vi "CubeLiftOutput.vi"   [LabVIEW 2017]
uses:
  CubeLiftOutput.ctl
  <vilib>/Rock Robotics/WPI/ThirdParty/Phoenix-LabVIEW/Motor Controller/Controls/CTRE_Phoenix_MotorControl_ControlMode.ctl
  <vilib>/Rock Robotics/WPI/Solenoid/WPI_SolenoidValue.ctl
  <vilib>/Rock Robotics/WPI/Solenoid/WPI_SolenoidSetEnum.vi
types:
  T1 = typedef "CubeLiftOutput.ctl" = cluster{"LiftOutputSetting":dbl, "DepositCube?":bool, "LiftControlMode":T2}
  T2 = typedef "CTRE_Phoenix_MotorControl_ControlMode.ctl" = u16
  T3 = typedef "WPI_SolenoidValue.ctl" = enum16{"Off", "On", "Forward", "Reverse"}
  T4 = typedef "WPI_MotorControlDeviceRef.ctl" = cluster{"DeviceStatus":errorcluster, "Type":T5, "PWM":cluster{"PWM Channel":T6, "DeadBand":T7}, "CAN":cluster{"Device Number":u8, "SetOutput VI Ref":variant, "GetOutput VI Ref":variant, "Enable VI Ref":variant, "Disable VI Ref":variant, "Data":variant}, "Invert":bool, "DIO PWM":cluster{"PWM \"Enable\" Channel":T6, "DIOChannel":T8, "PWM Rate":dbl}}
  T5 = typedef "WPI_MotorControlType.ctl" = enum16{"PWM", "CAN", "DIO PWM"}
  T6 = typedef "FPGA_DIOPWMChannel.ctl" = enum8{"PWM 0", "PWM 1", "PWM 2", "PWM 3", "PWM 4", "PWM 5", "PWM 6", "PWM 7", "PWM 8", "PWM 9", "PWM MXP 0", "PWM MXP 1", "PWM MXP 2", "PWM MXP 3", "PWM MXP 4", "PWM MXP 5", "PWM MXP 6", "PWM MXP 7", "PWM MXP 8", "PWM MXP 9", "Invalid"}
  T7 = typedef "WPI_PWMDeadband.ctl" = cluster{"Name":string, "maxPositivePwm":i32, "minPositivePwm":i32, "centerPwm":i32, "maxNegativePwm":i32, "minNegativePwm":i32, "angularRange":u16}
  T8 = typedef "FPGA_DIOChannel.ctl" = enum8{"DIO 0", "DIO 1", "DIO 2", "DIO 3", "DIO 4", "DIO 5", "DIO 6", "DIO 7", "DIO 8", "DIO 9", "DIO MXP 0", "DIO MXP 1", "DIO MXP 2", "DIO MXP 3", "DIO MXP 4", "DIO MXP 5", "DIO MXP 6", "DIO MXP 7", "DIO MXP 8", "DIO MXP 9", "DIO MXP 10", "DIO MXP 11", "DIO MXP 12", "DIO MXP 13", "DIO MXP 14", "DIO MXP 15", "SPI Port CS1", "SPI Port CS2", "SPI Port CS3", "SPI Port MISO", "SPI Port MOSI", "Invalid"}
  T9 = typedef "WPI_SolenoidDevRef.ctl" = cluster{"DevStatus":errorcluster, "Pneumatics Control Module":u8, "Forward Solenoid Channel":T10, "Reverse Solenoid Channel":T10}
  T10 = typedef "WPI_SolenoidChannel.ctl" = enum8{"Solenoid 0", "Solenoid 1", "Solenoid 2", "Solenoid 3", "Solenoid 4", "Solenoid 5", "Solenoid 6", "Solenoid 7", "Invalid"}
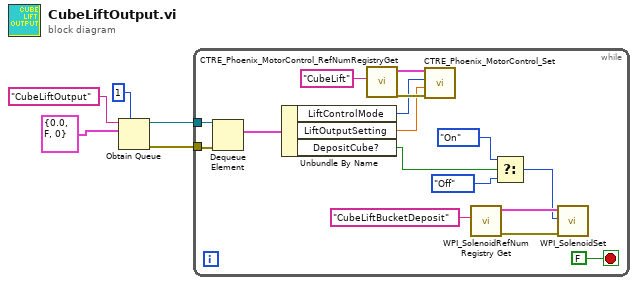
[diagram p0: block diagram]
diagram:
  n1 = Obtain Queue(max queue size (-1, unlimited)=1, name (unnamed)="CubeLiftOutput", element data type=T1 {"LiftOutputSetting"=0.0, "DepositCube?"=FALSE, "LiftControlMode"=0} ("CubeLiftOutput")) -> (queue out=w1:refnum<queue>, error out=w3:errorcluster)  [unwired: 2 in, 1 out]
  n2 = while {
    tunnel: w3 -> [w10]
    tunnel: w1 -> [w11]
    stop <- FALSE stop-if-true
    n3 = Dequeue Element(queue=w11, error in (no error)=w10) -> (element=w9:T1)  [unwired: 1 in, 3 out]
    n4 = Unbundle By Name(w9) -> ("LiftControlMode"=w6:T2, "LiftOutputSetting"=w7:dbl, "DepositCube?"=w8:bool)
    n5 = call <vilib>:"CTRE_Phoenix_MotorControl_RefNumRegistryGet.vi"("refnum name"="CubeLift") -> ("error out"=w12:errorcluster, "PhoenixMotorControlDevRef"=w13:T4)  [unwired: 9 in]
    n6 = call <vilib>:"CTRE_Phoenix_MotorControl_Set.vi"("error in (no error)"=w12, "Output"=w7, "Control Mode"=w6, "PhoenixMotorControlDevRef"=w13) -> ()  [unwired: 6 in, 2 out]
    n7 = call <vilib>:"WPI_SolenoidRefNum Registry Get.vi"("refnum name"="CubeLiftBucketDeposit") -> ("error out"=w19:errorcluster, "SolenoidDevRef"=w17:T9)  [unwired: 9 in]
    n8 = Select(t=WPI_SolenoidValue."On", s=w8, f=WPI_SolenoidValue."Off" ("Value")) -> (s? t:f=w14:T3)
    n9 = call-poly <vilib>:"WPI_SolenoidSet.vi"("error in (no error)"=w19, "Value"=w14, "SolenoidDevRef"=w17) -> ()  [unwired: 7 in, 2 out]
  }
